vi "Teleop.vi"(10 "Match Info":T1={"Autonomous Elapsed Seconds"=0.0, "TeleOp Elapsed Seconds"=0.0, "Disabled Elapsed Seconds"=0.0, "Visited Autonomous"=FALSE, "Visited TeleOp"=FALSE, "Visited Disabled"=FALSE, "Autonomous Settings"={"Autonomous Style"=enum."Independent", "VI Refnum"=refnum}}, 11 "Call Context":T2) -> ()   [LabVIEW 2018]
doc: "This VI is called for each enabled TeleOp packet received from the DS. It is typically used to read from joysticks and other inputs and update I/O or setpoints for timed control loops. It should complete and return within 20 milliseconds or risk missing DS packets."
uses:
  <vilib>/Rock Robotics/WPI/DriverStation/WPI_DriverStationDerivedRobotMode.ctl
  <vilib>/Rock Robotics/WPI/DriverStation/WPI_DriverStationMatch Info.ctl
  <vilib>/Rock Robotics/WPI/Solenoid/WPI_SolenoidValue.ctl
  Framework/Robot Global Data.vi
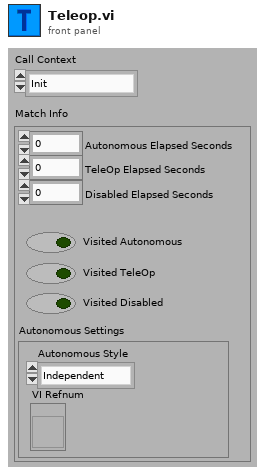
[diagram p1: front panel]
types:
  T1 = typedef "WPI_DriverStationMatch Info.ctl" = cluster{"Autonomous Elapsed Seconds":dbl, "TeleOp Elapsed Seconds":dbl, "Disabled Elapsed Seconds":dbl, "Visited Autonomous":bool, "Visited TeleOp":bool, "Visited Disabled":bool, "Autonomous Settings":cluster{"Autonomous Style":enum16{"Iterative", "Independent"}, "VI Refnum":refnum<vi>}}
  T2 = typedef "WPI_DriverStationDerivedRobotMode.ctl" = enum16{"Init", "Execute", "Stop"}
  T3 = typedef "Command Status Info.ctl" = cluster{"Name":string, "Status":T4, "notifier out":T5}
  T4 = typedef "Completion Status.ctl" = enum16{"Successful", "Aborted", "Incomplete"}
  T5 = typedef "Completion Notifier.ctl" = refnum<notifier>
  T6 = typedef "WPI_SolenoidValue.ctl" = enum16{"Off", "On", "Forward", "Reverse"}
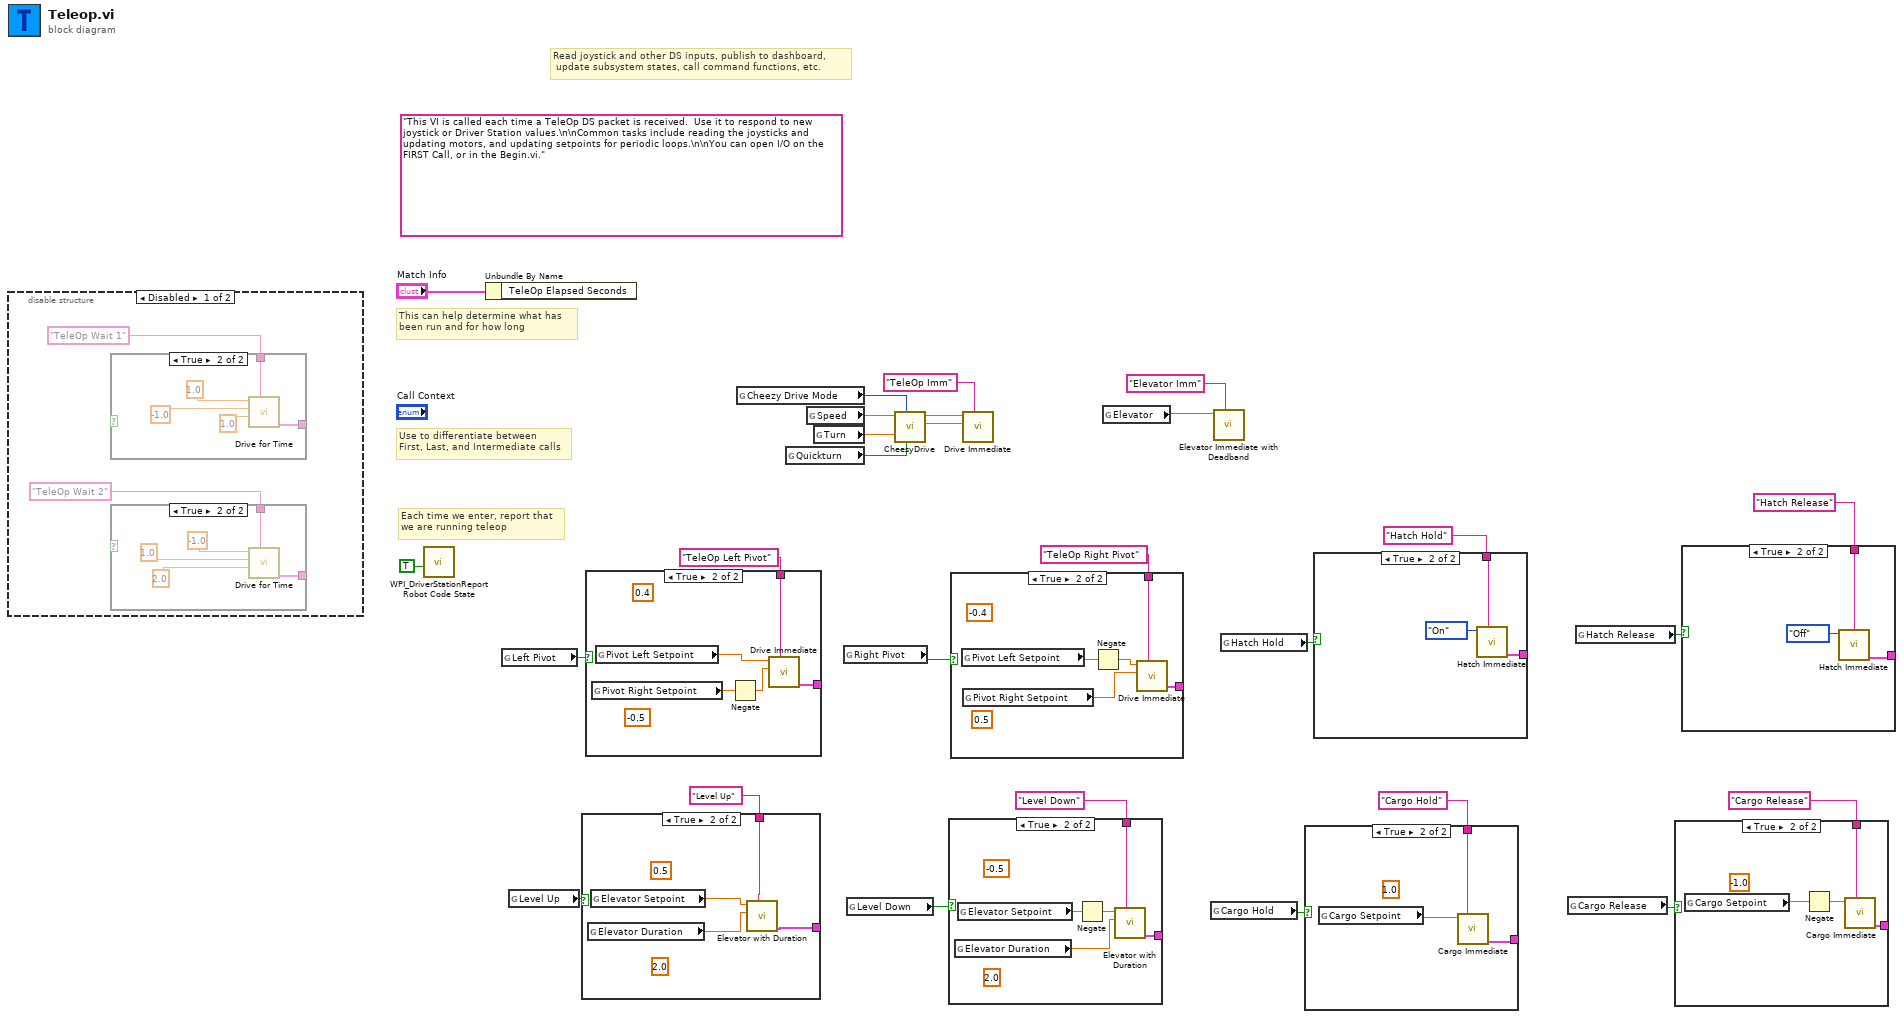
[diagram p0: block diagram]
diagram:
  (unwired) "This VI is called each time a TeleOp DS packet is received.  Use it to respond to new joystick or Driver Station values.\n\nCommon tasks include reading the joysticks and updating motors, and updating setpoints for periodic loops.\n\nYou can open I/O on the FIRST Call, or in the Begin.vi."
  # "Read joystick and other DS inputs, publish to dashboard,\n update subsystem states, call command functions, etc."
  # "Each time we enter, report that\nwe are running teleop"
  # "Use to differentiate between\nFirst, Last, and Intermediate calls"
  # "This can help determine what has\nbeen run and for how long"
  n1 = disable-structure shown="Disabled" {
    frame Disabled {
      n2 = case shown="True" w29 {
        tunnel: [_ w40] -> _
        tunnel: "TeleOp Wait 1" ("Description") -> [_ w39]
        frame False {
        }
        frame True {
          n3 = call "Drive for Time.vi"("Description"=w39, "Seconds"=1.0, "Right Speed"=-1.0, "Left Speed"=1.0) -> ("Command Info Out"=w40:T3)  [unwired: 7 in]
        }
      }
      n4 = case shown="True" w28 {
        tunnel: [_ w34] -> _
        tunnel: "TeleOp Wait 2" ("Description") -> [_ w33]
        frame False {
        }
        frame True {
          n5 = call "Drive for Time.vi"("Description"=w33, "Seconds"=2.0, "Right Speed"=1.0, "Left Speed"=-1.0) -> ("Command Info Out"=w34:T3)  [unwired: 7 in]
        }
      }
    }
    frame Enabled {
    }
  }
  n6 = call <vilib>:"WPI_DriverStationReport Robot Code State.vi"("TeleOp"=TRUE ("Autonomous")) -> ()  [unwired: 10 in, 1 out]
  n7 = Unbundle By Name("Match Info") -> ()  [unwired: 1 out]
  n8 = global read "Robot Global Data.vi" "Left Pivot"() -> (w16:bool)
  n9 = global read "Robot Global Data.vi" "Level Up"() -> (w13:bool)
  n10 = case shown="True" w13 {
    tunnel: [_ w45] -> _
    tunnel: "Level Up" ("Description") -> [_ w44]
    frame False {
    }
    frame True {
      (unwired) 2.0 ("Duration (s)")
      (unwired) 0.5 ("Setpoint")
      n11 = global read "Robot Global Data.vi" "Elevator Duration"() -> (w42:dbl)
      n12 = global read "Robot Global Data.vi" "Elevator Setpoint"() -> (w43:dbl)
      n13 = call "Elevator with Duration.vi"("Description"=w44, "Duration (s)"=w42, "Setpoint"=w43) -> ("Command Info Out"=w45:T3)  [unwired: 8 in]
    }
  }
  n14 = case shown="True" w16 {
    tunnel: [_ w50] -> _
    tunnel: "TeleOp Left Pivot" ("Description") -> [_ w49]
    frame False {
    }
    frame True {
      (unwired) -0.5 ("Right Setpoint")
      (unwired) 0.4 ("Left Setpoint")
      n15 = global read "Robot Global Data.vi" "Pivot Right Setpoint"() -> (w47:dbl)
      n16 = global read "Robot Global Data.vi" "Pivot Left Setpoint"() -> (w48:dbl)
      n17 = Negate(x=w47) -> (-x=w46:dbl)
      n18 = call "Drive Immediate.vi"("Description"=w49, "Right Setpoint"=w46, "Left Setpoint"=w48) -> ("Command Info Out"=w50:T3)  [unwired: 8 in]
    }
  }
  n19 = global read "Robot Global Data.vi" "Cheezy Drive Mode"() -> (w1:u32)
  n20 = global read "Robot Global Data.vi" "Quickturn"() -> (w20:bool)
  n21 = global read "Robot Global Data.vi" "Speed"() -> (w22:dbl)
  n22 = global read "Robot Global Data.vi" "Turn"() -> (w21:dbl)
  n23 = global read "Robot Global Data.vi" "Right Pivot"() -> (w17:bool)
  n24 = global read "Robot Global Data.vi" "Level Down"() -> (w12:bool)
  n25 = call "CheesyDrive.vi"("Quickturn"=w20, "SlowMode"=w1, "Wheel"=w21, "Throttle"=w22) -> ("Right PWM"=w23:dbl, "Left PWM"=w24:dbl)  [unwired: 6 in]
  n26 = case shown="True" w12 {
    tunnel: "Level Down" ("Description") -> [_ w55]
    tunnel: [_ w54] -> _
    frame False {
    }
    frame True {
      (unwired) 2.0 ("Duration (s)")
      (unwired) -0.5 ("Setpoint")
      n27 = global read "Robot Global Data.vi" "Elevator Duration"() -> (w52:dbl)
      n28 = global read "Robot Global Data.vi" "Elevator Setpoint"() -> (w53:dbl)
      n29 = Negate(x=w53) -> (-x=w51:dbl)
      n30 = call "Elevator with Duration.vi"("Description"=w55, "Duration (s)"=w52, "Setpoint"=w51) -> ("Command Info Out"=w54:T3)  [unwired: 8 in]
    }
  }
  n31 = case shown="True" w17 {
    tunnel: [_ w60] -> _
    tunnel: "TeleOp Right Pivot" ("Description") -> [_ w59]
    frame False {
    }
    frame True {
      (unwired) 0.5 ("Right Setpoint")
      (unwired) -0.4 ("Left Setpoint")
      n32 = global read "Robot Global Data.vi" "Pivot Left Setpoint"() -> (w57:dbl)
      n33 = global read "Robot Global Data.vi" "Pivot Right Setpoint"() -> (w58:dbl)
      n34 = Negate(x=w57) -> (-x=w56:dbl)
      n35 = call "Drive Immediate.vi"("Description"=w59, "Right Setpoint"=w58, "Left Setpoint"=w56) -> ("Command Info Out"=w60:T3)  [unwired: 8 in]
    }
  }
  n36 = call "Drive Immediate.vi"("Description"="TeleOp Imm", "Right Setpoint"=w23, "Left Setpoint"=w24) -> ()  [unwired: 8 in, 1 out]
  n37 = global read "Robot Global Data.vi" "Elevator"() -> (w7:dbl)
  n38 = global read "Robot Global Data.vi" "Cargo Hold"() -> (w9:bool)
  n39 = call "Elevator Immediate with Deadband.vi"("Description"="Elevator Imm", "Setpoint"=w7) -> ()  [unwired: 9 in, 1 out]
  n40 = global read "Robot Global Data.vi" "Hatch Hold"() -> (w2:bool)
  n41 = case shown="True" w9 {
    tunnel: [_ w63] -> _
    tunnel: "Cargo Hold" ("Description") -> [_ w62]
    frame False {
    }
    frame True {
      (unwired) 1.0 ("Left Setpoint")
      n42 = global read "Robot Global Data.vi" "Cargo Setpoint"() -> (w61:dbl)
      n43 = call "Cargo Immediate.vi"("Description"=w62, "Setpoint"=w61) -> ("Command Info Out"=w63:T3)  [unwired: 9 in]
    }
  }
  n44 = case shown="True" w2 {
    tunnel: "Hatch Hold" ("Description") -> [_ w66]
    tunnel: [_ w65] -> _
    frame False {
    }
    frame True {
      n45 = call "Hatch Immediate.vi"("Description"=w66, "Hatch Action"=WPI_SolenoidValue."On") -> ("Command Info Out"=w65:T3)  [unwired: 9 in]
    }
  }
  n46 = global read "Robot Global Data.vi" "Cargo Release"() -> (w8:bool)
  n47 = global read "Robot Global Data.vi" "Hatch Release"() -> (w3:bool)
  n48 = case shown="True" w8 {
    tunnel: [_ w70] -> _
    tunnel: "Cargo Release" ("Description") -> [_ w69]
    frame False {
    }
    frame True {
      (unwired) -1.0 ("Left Setpoint")
      n49 = global read "Robot Global Data.vi" "Cargo Setpoint"() -> (w68:dbl)
      n50 = Negate(x=w68) -> (-x=w67:dbl)
      n51 = call "Cargo Immediate.vi"("Description"=w69, "Setpoint"=w67) -> ("Command Info Out"=w70:T3)  [unwired: 9 in]
    }
  }
  n52 = case shown="True" w3 {
    tunnel: "Hatch Release" ("Description") -> [_ w73]
    tunnel: [_ w72] -> _
    frame False {
    }
    frame True {
      n53 = call "Hatch Immediate.vi"("Description"=w73, "Hatch Action"=WPI_SolenoidValue."Off") -> ("Command Info Out"=w72:T3)  [unwired: 9 in]
    }
  }
